vi "LCD Set Cursor Mode.vi"(0 "Arduino Resource":T1, 5 "Cursor On? (T)":bool=TRUE, 7 "Cursor Blink? (F)":bool, 11 "error out":errorcluster) -> (4 "Arduino Resource":T1, 15 "error out":errorcluster)   [LabVIEW 2015, in "LabVIEW Interface for Arduino.lvlib"]
doc: "Sets the properties for the cursor on the LCD Screen. The visibility and the blinking property of the cursor can be enabled or disabled."
uses:
  <vilib>/LabVIEW Interface for Arduino/LabVIEW Interface for Arduino.lvlib
  <vilib>/LabVIEW Interface for Arduino/Type Defs/Arduino Resource.ctl
  <vilib>/LabVIEW Interface for Arduino/Type Defs/Board Type.ctl
  <vilib>/LabVIEW Interface for Arduino/Type Defs/Command.ctl
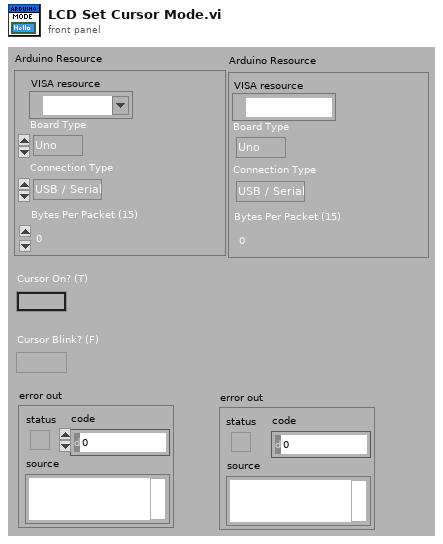
[diagram p1: front panel]
types:
  T1 = typedef "LabVIEW Interface for Arduino.lvlib/Arduino Resource.ctl" = cluster{"VISA resource":refnum<visa-resource-name>, "Board Type":T2, "Connection Type":enum8{"USB / Serial"}, "Bytes Per Packet (15)":u8}
  T2 = typedef "LabVIEW Interface for Arduino.lvlib/Board Type.ctl" = enum16{"Uno", "Dimuelanove w/Atmega 328", "Mega 2560"}
  T3 = typedef "LabVIEW Interface for Arduino.lvlib/Command.ctl" = enum8{"setArduinoMode", "flushSerial", "setPinMode", "digitalWritePin", "digitalWritePort", "tone", "digitalReadPin", "digitalReadPort", "analogReadPin", "analogReadPort", "pwmWritePin", "pwmWritePort", "sevenSegment_Configure", "sevenSegment_Write", "I2C Init", "I2C Write", "I2C Read", "SPI Init", "SPI Set Bit Order", "SPI Set Clock Divider", "SPI Set Data Mode", "SPI Send / Receive", "SPI Close", "Servo Set Num Servos", "Servo Config Servo", "Servo Write Angle", "Servo Read Angle", "Servo Write Pulse Width", "Servo Read Pulse Width", "Servo Detach", "LCD Init", "LCD Set Size", "LCD Set Cursor Mode", "LCD Clear", "LCD Set Cursor Position", "LCD Print", "LCD Display Power", "LCD Scroll Display", "LCD Autoscroll", "LCD Print Direction", "LCD Create Custom Char", "LCD Print Custom Char", "contAcqOn", "contAcqOff", "getFirmwareVersion", "FiniteSampleStart"}
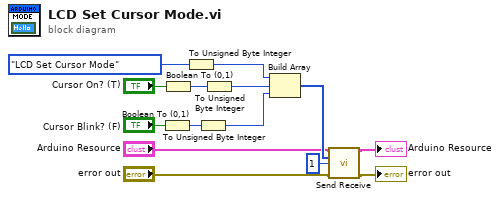
[diagram p0: block diagram]
diagram:
  n1 = Boolean To (0,1)(Boolean="Cursor Blink? (F)") -> (0, 1=w1:i16)
  n2 = Boolean To (0,1)(Boolean="Cursor On? (T)") -> (0, 1=w2:i16)
  n3 = To Unsigned Byte Integer(number=Command."LCD Set Cursor Mode" ("Command")) -> (unsigned 8bit integer=w8:u8)
  n4 = To Unsigned Byte Integer(number=w1) -> (unsigned 8bit integer=w6:u8)
  n5 = To Unsigned Byte Integer(number=w2) -> (unsigned 8bit integer=w5:u8)
  n6 = Build Array(w8, w5, w6) -> (w13:u8[])
  n7 = call <vilib>:"Send Receive.vi"("Arduino Resource"="Arduino Resource", "Data"=w13, "Bytes To Read (0)"=u8 1, "error in"="error out") -> ("Arduino Resource"=→"Arduino Resource":T1, "error out"=→"error out":errorcluster)  [unwired: 9 in, 1 out]
